vi "Read Trace Data.vi"(6 "Trace Data Size (0)":i32, 7 "Trace Data Offset (0)":i32, 8 "error in (no error)":errorcluster, 9 "Measurement Type (0: Current)":i32(ring) items=["Current", "Limit", "Math", "Resistance", "Voltage"], 10 "Channel (1: Channel 1)":i32(ring)=1 items=["Channel 1"=1, "Channel 2"=2], 11 "VISA resource name":refnum<visa-resource-name>) -> (0 "error out":errorcluster, 2 "Trace Buffer Data":dbl, 3 "VISA resource name out":refnum<visa-resource-name>)   [LabVIEW 2012, in "Keysight B2980 Series.lvlib"]
doc: "Returns specified measurement data in the trace buffer."
uses:
  Keysight B2980 Series.lvlib
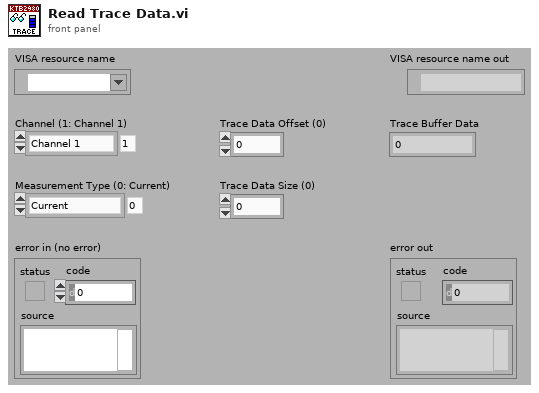
[diagram p1: front panel]
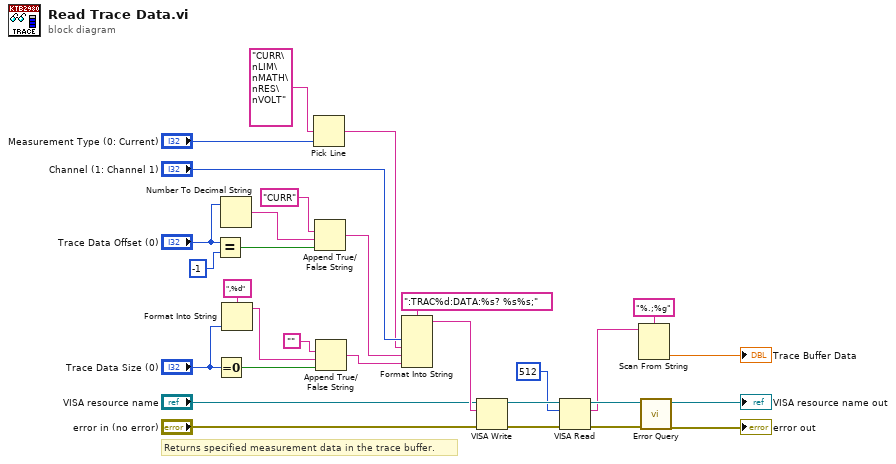
[diagram p0: block diagram]
diagram:
  # "Returns specified measurement data in the trace buffer."
  n1 = Equal?(x="Trace Data Offset (0)", y=-1) -> (x = y?=w10:bool)
  n2 = Equal To 0?(x="Trace Data Size (0)") -> (x = 0?=w4:bool)
  n3 = Number To Decimal String(number="Trace Data Offset (0)") -> (decimal integer string=w8:string)  [unwired: 1 out]
  n4 = Format Into String(format string=",%d", "Trace Data Size (0)") -> (resulting string=w5:string)  [unwired: 2 in, 1 out]
  n5 = Pick Line(multi-line string="CURR\nLIM\nMATH\nRES\nVOLT", line index="Measurement Type (0: Current)") -> (output string=w26:string)  [unwired: 1 out]
  n6 = Append True/False String(1:w10, 2:w8, 3:"CURR") -> (0:w7:string)  [unwired: 1 in]
  n7 = Append True/False String(1:w4, 2:w5, 3:"") -> (0:w3:string)  [unwired: 1 in]
  n8 = Format Into String(format string=":TRAC%d:DATA:%s? %s%s;", "Channel (1: Channel 1)", w26, w7, w3) -> (resulting string=w25:string)  [unwired: 2 in, 1 out]
  n9 = VISA Write(VISA resource name="VISA resource name", write buffer=w25, error in (no error)="error in (no error)") -> (VISA resource name out=w18:refnum<visa-resource-name>, error out=w17:errorcluster)  [unwired: 1 out]
  n10 = VISA Read(VISA resource name=w18, byte count=u32 512, error in (no error)=w17) -> (VISA resource name out=w16:refnum<visa-resource-name>, read buffer=w13:string, error out=w15:errorcluster)  [unwired: 1 out]
  n11 = Scan From String(format string="%.;%g", input string=w13) -> (output 1=→"Trace Buffer Data":dbl)  [unwired: 2 in, 4 out]
  n12 = call "Error Query.vi"("error in (no error)"=w15, "VISA resource name"=w16) -> ("error out"=→"error out":errorcluster, "VISA resource name out"=→"VISA resource name out":refnum<visa-resource-name>)  [unwired: 8 out]
